vi "Rename Channel Name List.vi"(7 "delete (T)":bool, 9 "Enter New Name":string, 10 "Choose Channel names":string(combo), 11 "Cluster in":T1) -> (1 "dialog":string, 3 "Cluster out":T1)   [LabVIEW 2020]
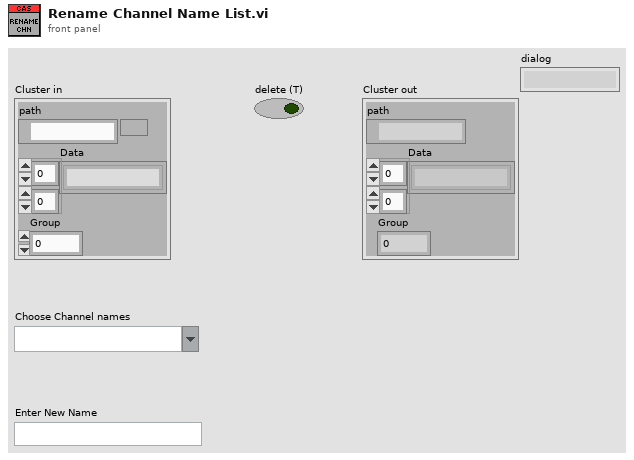
[diagram p1: front panel]
types:
  T1 = cluster{"path":path, "Data":string[][], "Group":i32}
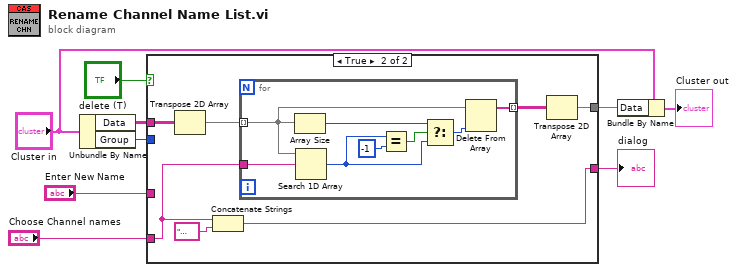
[diagram p0: block diagram]
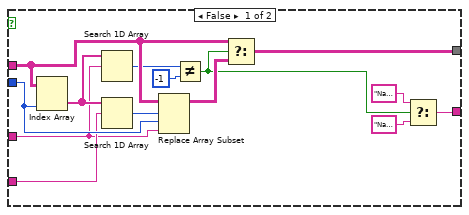
[diagram p2: hidden frame]
diagram:
  n1 = Unbundle By Name("Cluster in") -> ("Data"=w9:string[][], "Group"=w7:i32)
  n2 = case shown="True" "delete (T)" {
    tunnel: w9 -> [w22 w30]
    tunnel: [w21 w27] -> w8
    tunnel: w7 -> [w16 _]
    tunnel: "Choose Channel names" -> [w15 w26]
    tunnel: "Enter New Name" -> [w14 _]
    tunnel: [w10 w24] -> w1
    frame False {
      n3 = Index Array(array=w22, index (col)=w16) -> (element=w18:string[])  [unwired: 1 in]
      n4 = Search 1D Array(1D array=w18, element=w14) -> (index of element=w19:i32)  [unwired: 1 in]
      n5 = Search 1D Array(1D array=w18, element=w15) -> (index of element=w17:i32)  [unwired: 1 in]
      n6 = Replace Array Subset(array=w22, new element=w14, index (row)=w17, index (col)=w16) -> (w23:string[][])
      n7 = Not Equal?(x=w19, y=-1) -> (x != y?=w11:bool)
      n8 = Select(t=w22, s=w11, f=w23) -> (s? t:f=w21:string[][])
      n9 = Select(t="Name You Entered is already Exist!" ("message"), s=w11, f="Name Successfully Changed.") -> (s? t:f=w10:string)
    }
    frame True {
      n10 = Transpose 2D Array(2D array=w30) -> (transposed array=w28:string[][])
      n11 = Concatenate Strings(w26, " Deleted Successfully." ("string")) -> (w24:string)
      n12 = for {
        tunnel: w28 -> [w35] mode=indexing
        tunnel: [w37] -> w29 mode=indexing
        tunnel: w26 -> [w36]
        n13 = Array Size(array=w35) -> (size(s)=w34:i32)
        n14 = Search 1D Array(1D array=w35, element=w36) -> (index of element=w32:i32)  [unwired: 1 in]
        n15 = Equal?(x=w32, y=-1 ("index of element")) -> (x = y?=w33:bool)
        n16 = Select(t=w34, s=w33, f=w32) -> (s? t:f=w31:i32)
        n17 = Delete From Array(array=w35, index=w31) -> (array with subset deleted=w37:string[])  [unwired: 1 in, 1 out]
      }
      n18 = Transpose 2D Array(2D array=w29) -> (transposed array=w27:string[][])
    }
  }
  "dialog" <- w1
  n19 = Bundle By Name(cluster="Cluster in", "Data"=w8) -> (→"Cluster out":T1)
